vi "Autozero.vi"(0 "Vmin (V)":dbl, 1 "IFoffset (V)":dbl, 2 "Enable":bool, 3 "Max Gain":bool) -> ()   [LabVIEW 2018]
uses:
  Global 2.vi
panel:
  # "Adjusts offset to eliminate\npedestal drift"
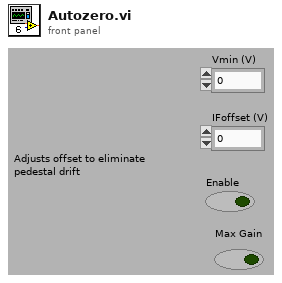
[diagram p1: front panel]
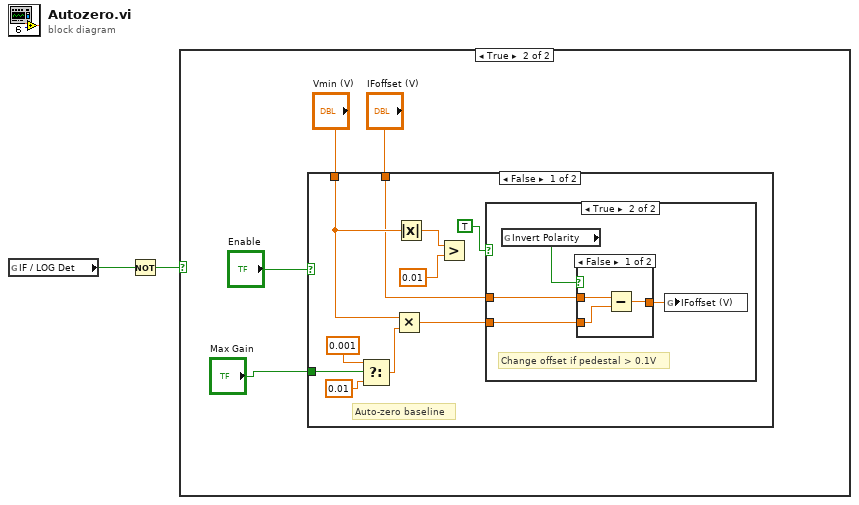
[diagram p0: block diagram]
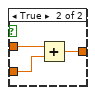
[diagram p4: hidden frame]
diagram:
  n1 = global read "Global 2.vi" "IF / LOG Det"() -> (w1:bool)
  n2 = Not(x=w1) -> (.not. x?=w2:bool)
  n3 = case shown="True" w2 {
    frame False {
    }
    frame True {
      n4 = case shown="False" "Enable" {
        tunnel: "Vmin (V)" -> [w14 _]
        tunnel: "IFoffset (V)" -> [w13 _]
        tunnel: "Max Gain" -> [w11 _]
        frame False {
          # "Auto-zero baseline"
          n5 = Select(t=0.001, s=w11, f=0.01) -> (s? t:f=w10:dbl)
          n6 = Multiply(x=w14, y=w10) -> (x*y=w12:dbl)
          n7 = Absolute Value(x=w14) -> (abs(x)=w15:dbl)
          n8 = Greater?(x=w15, y=0.01) -> ()  [unwired: 1 out]
          n9 = case shown="True" TRUE {
            tunnel: w12 -> [_ w20]
            tunnel: w13 -> [_ w19]
            frame False {
            }
            frame True {
              # "Change offset if pedestal > 0.1V"
              n10 = global read "Global 2.vi" "Invert Polarity"() -> (w17:bool)
              n11 = case shown="False" w17 {
                tunnel: w20 -> [w21 w26]
                tunnel: w19 -> [w22 w25]
                tunnel: [w23 w24] -> w18
                frame False {
                  n12 = Subtract(x=w22, y=w21) -> (x-y=w23:dbl)
                }
                frame True {
                  n13 = Add(x=w25, y=w26) -> (x+y=w24:dbl)
                }
              }
              n14 = global write "Global 2.vi" "IFoffset (V)"(w18) -> ()
            }
          }
        }
        frame True {
        }
      }
    }
  }
